vi "SensorInterrupt.vi"(8 "error in (no error)":errorcluster, 11 "Intake in":refnum<class "Intake.lvclass">) -> (0 "error out":errorcluster, 3 "Intake out":refnum<class "Intake.lvclass">)   [LabVIEW 2017, in "Intake.lvclass"]
uses:
  Intake.lvclass
  Subsystem.lvclass
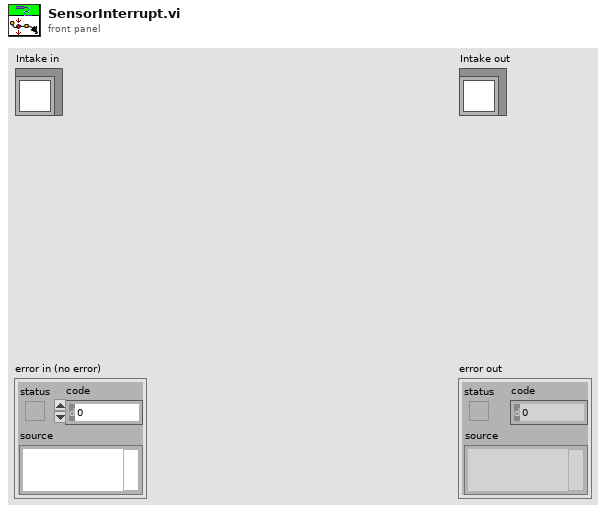
[diagram p1: front panel]
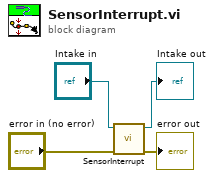
[diagram p0: block diagram]
diagram:
  n1 = call-parent "SensorInterrupt.vi"("error in (no error)"="error in (no error)", "Subsystem in"="Intake in") -> ("error out"=→"error out":errorcluster, "Subsystem out"=→"Intake out":refnum<class "Intake.lvclass">)  [unwired: 8 in]
